vi "4.7.vi"() -> ()   [LabVIEW 2017]
panel:
  out "随机数":i32
  out "输入值":i32
  out "次数":i32
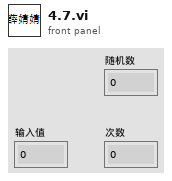
[diagram p1: front panel]
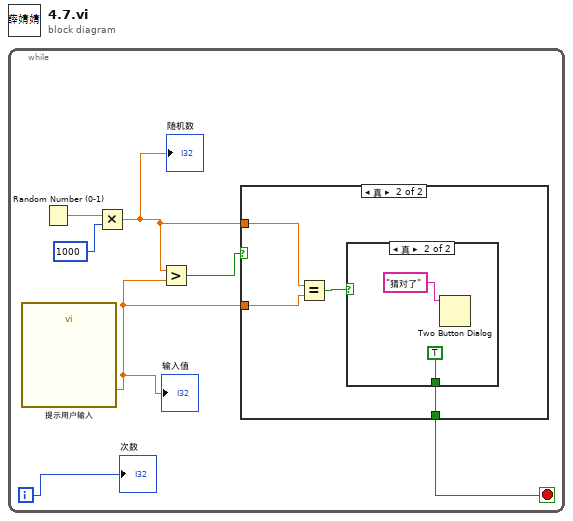
[diagram p0: block diagram]
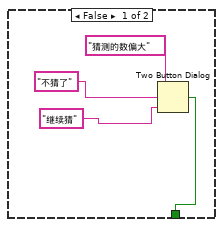
[diagram p2: hidden frame]
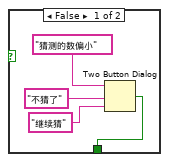
[diagram p3: hidden frame]
diagram:
  n1 = while {
    i -> [w3]
    stop <- w4 stop-if-true
    n2 = call "提示用户输入"() -> ("请在1-1000猜"=w2:dbl)  [unwired: 17 in, 2 out]
    "输入值" <- w2
    n3 = Random Number (0-1)() -> (number: 0 to 1=w7:dbl)
    n4 = Multiply(x=w7, y=1000) -> (x*y=w1:dbl)
    "随机数" <- w1
    n5 = Greater?(x=w1, y=w2) -> (0:w5:bool)
    n6 = case shown="真" w5 {
      tunnel: w2 -> [_ w15]
      tunnel: w1 -> [_ w14]
      tunnel: [w10 w12] -> w4
      frame False {
        n7 = Two Button Dialog(message="猜测的数偏大", 1:"继续猜", 2:"不猜了") -> (T button?=w10:bool)
      }
      frame True {
        n8 = Equal?(x=w14, y=w15) -> (x = y?=w13:bool)
        n9 = case shown="真" w13 {
          tunnel: [w18 TRUE] -> w12
          frame False {
            n10 = Two Button Dialog(message="猜测的数偏小", 1:"继续猜", 2:"不猜了") -> (T button?=w18:bool)
          }
          frame True {
            n11 = Two Button Dialog(message="猜对了") -> ()  [unwired: 2 in, 1 out]
          }
        }
      }
    }
    "次数" <- w3
  }
